vi "CAN_init.vi"(9 "Selected Count":i32, 10 "error in (no error)":errorcluster, 11 "DEVICE CONFIG":T2(array[cluster])=[{"DeviceIndex"=0, "Mode"=1, "BaudRate"=500000, "DataBitRate"=0}]) -> (2 "error out":errorcluster, 3 "Device Handler":i64[](array[numeric]))   [LabVIEW 2026]
uses:
  <vilib>/Utility/importsl/GetValueByPointer/GetValueByPointer.xnode
  Include/DEVICE_CONFIG.ctl
  <vilib>/Utility/importsl/GetValueByPointer/datatype.ctl
panel:
  in  "Device Config":T1={"Handle"=[0, 0, 0, 0], "osRead"=[0, 0, 0, 0, 0], " osWrite"=[0, 0, 0, 0, 0], "Device Path 2"=[0, 1, 2, 3, 4, 5, 6, 7, 8, 9, 10, 11, 12, 13, 14, 15, 16, 17, 18, 19, 20, 21, 22, 23, 24, 25, 26, 27, 28, 0, 1, 2, 1, 2, 1, 1, 1, 0, 1, 0, 0, 0, 0, 0, 0, 0, 0, 0, 0, 0, 0, 0, 0, 0, 0, 1, 0, 0, 0, 0, 0, 0, 0, 0, 0, 0, 0, 0, 0, 0, 0, 0, 0, 0, 0, 0, 0, 0, 0, 0, 0, 0, 0, 0, 0, 0, 0, 0, 0, 0, 0, 0, 0, 0, 0, 0, 0, 0, 0, 0, 0, 0, 0, 0, 0, 0, 0, 0, 0, 0, 0, 0, 0, 0, 0, 0, 0, 0, 0, 0, 0, 0, 0, 0, 0, 0, 0, 0, 0, 0, 0, 0, 0, 0, 0, 0, 0, 0, 0, 0, 0, 0, 0, 0, 0, 0, 0, 0, 0, 0, 0, 0, 0, 0, 0, 0, 0, 0, 0, 0, 0, 0, 0, 0, 0, 0, 0, 0, 0, 0, 0, 0, 0, 0, 0, 0, 0, 0, 0, 0, 0, 0, 0, 0, 0, 0, 0, 0, 0, 0, 0, 0, 0, 0, 0, 0, 0, 0, 0, 0, 0, 0, 0, 0, 0, 0, 0, 0, 0, 0, 0, 0, 0, 0, 0, 0, 0, 0, 0, 0, 0, 0, 0, 0, 0, 0, 0, 0, 0, 0, 0, 0, 0, 0, 0, 0, 0, 0, 0, 0, 0, 0, 0, 0, 0, 0, 0, 0, 0, 0, 0, 0, 0, 0, 0, 0], "Mode"=0, "Serial Number 2"=0, "Keep Alive Received"=0, "Device Index"=0}
  out "CAN BaudRate":u8
  out "Device Handler":T3(array[cluster])
  out "CanFD Bitrate":u8
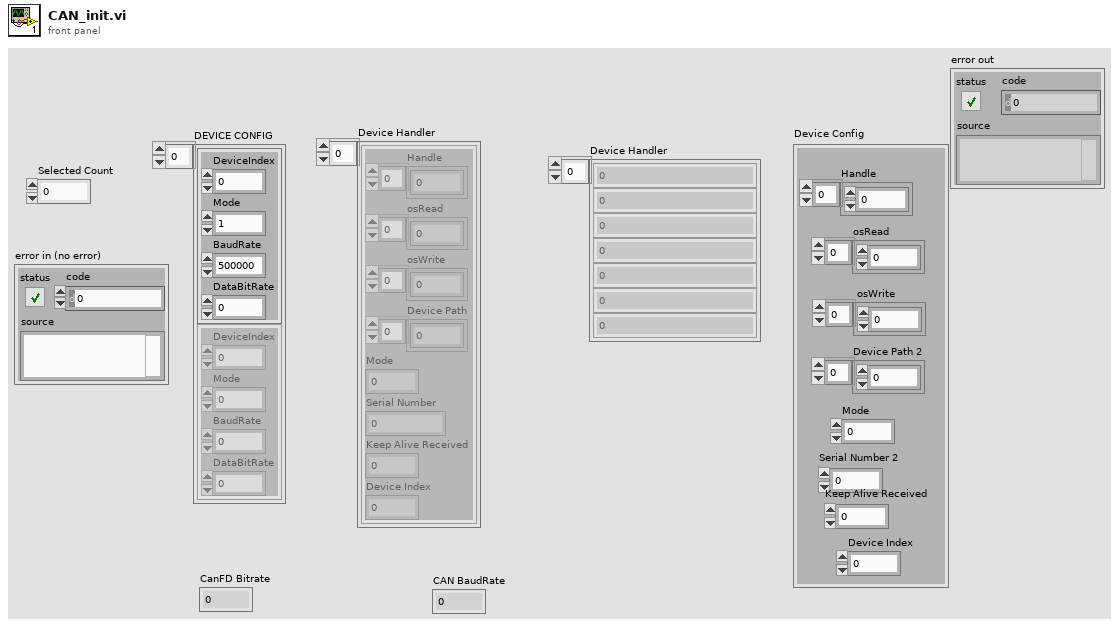
[diagram p1: front panel]
types:
  T1 = typedef "DEVICE_CONFIG.ctl" = cluster{"Handle":u8[], "osRead":u32[], " osWrite":u32[], "Device Path 2":u16[], "Mode":i32, "Serial Number 2":u32, "Keep Alive Received":u8, "Device Index":u8}
  T2 = cluster{"DeviceIndex":i32, "Mode":i32, "BaudRate":i32, "DataBitRate":i32}[]
  T3 = cluster{"Handle":u8[], "osRead":i32[], "osWrite":i32[], "Device Path":u16[], "Mode":i32, "Serial Number":u32, "Keep Alive Received":u8, "Device Index":u8}[]
  T4 = cluster{"DeviceIndex":i32, "Mode":i32, "BaudRate":i32, "DataBitRate":i32}
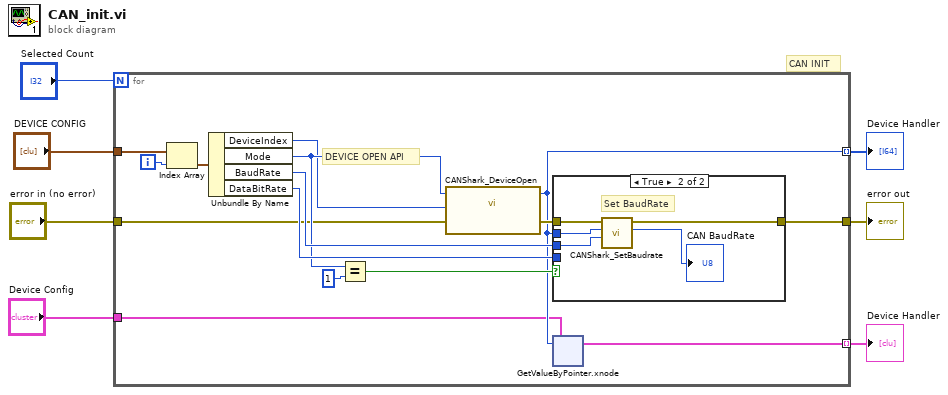
[diagram p0: block diagram]
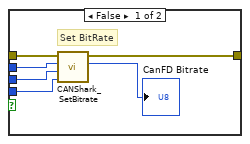
[diagram p2: hidden frame]
diagram:
  # "CAN INIT"
  n1 = for {
    N: "Selected Count" -> [_]
    tunnel: "DEVICE CONFIG" -> [w15]
    tunnel: [w16] -> w7 mode=indexing
    tunnel: [w13] -> w2 mode=indexing
    tunnel: "error in (no error)" -> [w10]
    tunnel: [w9] -> w4
    tunnel: "Device Config" -> [w8]
    i -> [w18]
    # "DEVICE OPEN API"
    n2 = Index Array(array=w15, index=w18) -> (element=w17:T4)
    n3 = Unbundle By Name(w17) -> ("DeviceIndex"=w11:i32, "Mode"=w12:i32, "BaudRate"=w20:i32, "DataBitRate"=w19:i32)
    n4 = Equal?(x=w12, y=1) -> (x = y?=w21:bool)
    n5 = call "CANShark_DeviceOpen.vi"("error in (no error)"=w10, "Device Index"=w11, "Mode"=w12) -> ("error out"=w14:errorcluster, "CANSHARK_DEVICE"=w13:i64)  [unwired: 7 in]
    n6 = case shown="True" w21 {
      tunnel: w20 -> [w23 w30]
      tunnel: w19 -> [w24 _]
      tunnel: w13 -> [w25 w31]
      tunnel: w14 -> [w26 w29]
      tunnel: [w28 w33] -> w9
      frame False {
        # "Set BitRate"
        n7 = call "CANShark_SetBitrate.vi"("Data Bitrate"=w24, "Nominal Bitrate"=w23, "Device Handler"=w25, "error in (no error)"=w26) -> ("CanFD Bitrate"=→"CanFD Bitrate":u8, "error out"=w28:errorcluster)  [unwired: 6 in]
      }
      frame True {
        # "Set BaudRate"
        n8 = call "CANShark_SetBaudrate.vi"("BaudRate"=w30, "Device Handler"=w31, "error in (no error)"=w29) -> ("CAN BaudRate"=→"CAN BaudRate":u8, "error out"=w33:errorcluster)  [unwired: 7 in]
      }
    }
    n9 = xnode "GetValueByPointer.xnode"("Pointer"=w13, "InputType"=w8) -> ("Output"=w16:T1)  [unwired: 2 in, 1 out]
  }
  "Device Handler" <- w7
  "error out" <- w4
  "Device Handler" <- w2
